vi "curvature to lookahead point.vi"(6 "Lookahead Distance":dbl, 11 "Path Data":T1={"Path"=[], "Target Velocities"=[], "Robot Location"=[], "Relative Robot Angle (rad)"=0.0, "Curvature"=0.0, "Lookahead Point"=[3064.399009129367, 18229.833030071386], "Lookahead Index"=8.422809037111724, "Closest Point"=[], "Closest Point Index"=0, "Left Velocity"=0.0, "Right Velocity"=0.0, "Left Encoder Vel"=0, "Right Encoder Vel"=0, "Left Encoder Pos"=0, "Right Encoder Pos"=0, "Inital Robot Angle (deg)"=0.0}) -> (3 "Path Data":T1={"Path"=[], "Target Velocities"=[], "Robot Location"=[], "Relative Robot Angle (rad)"=0.0, "Curvature"=0.0, "Lookahead Point"=[3064.399009129367, 18229.833030071386], "Lookahead Index"=8.422809037111724, "Closest Point"=[], "Closest Point Index"=0, "Left Velocity"=0.0, "Right Velocity"=0.0, "Left Encoder Vel"=0, "Right Encoder Vel"=0, "Left Encoder Pos"=0, "Right Encoder Pos"=0, "Inital Robot Angle (deg)"=0.0})   [LabVIEW 2018]
uses:
  path data.ctl
panel:
  out "Curvature":dbl
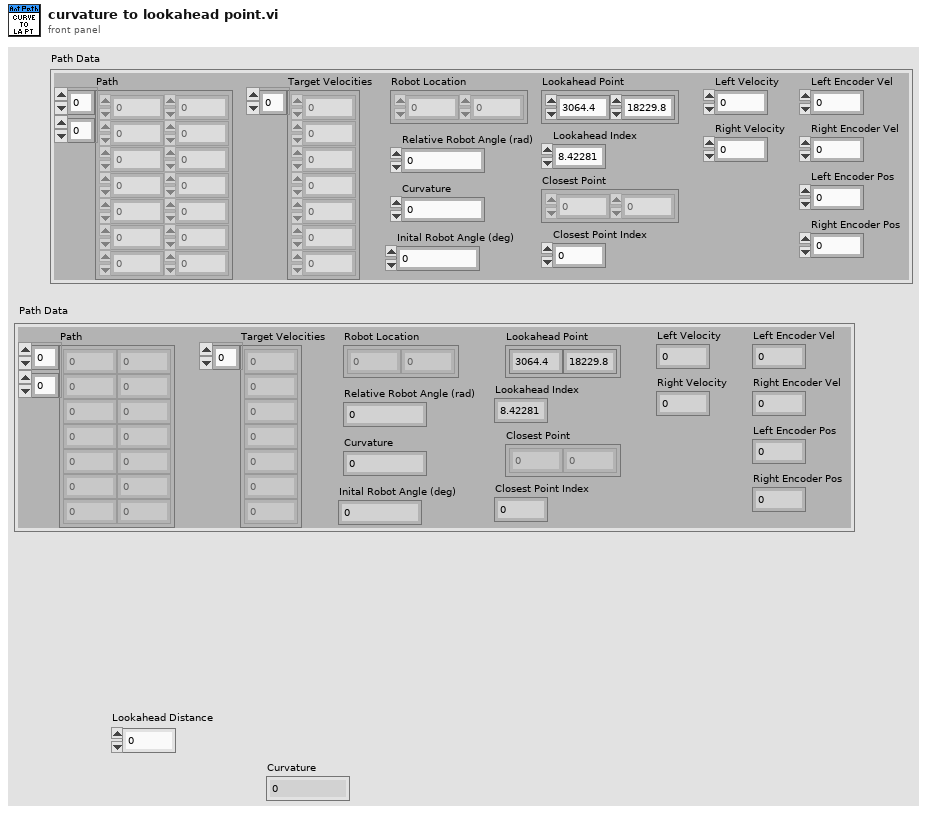
[diagram p1: front panel]
types:
  T1 = typedef "path data.ctl" = cluster{"Path":dbl[][], "Target Velocities":dbl[], "Robot Location":dbl[], "Relative Robot Angle (rad)":dbl, "Curvature":dbl, "Lookahead Point":dbl[], "Lookahead Index":dbl, "Closest Point":dbl[], "Closest Point Index":i32, "Left Velocity":dbl, "Right Velocity":dbl, "Left Encoder Vel":i32, "Right Encoder Vel":i32, "Left Encoder Pos":i32, "Right Encoder Pos":i32, "Inital Robot Angle (deg)":dbl}
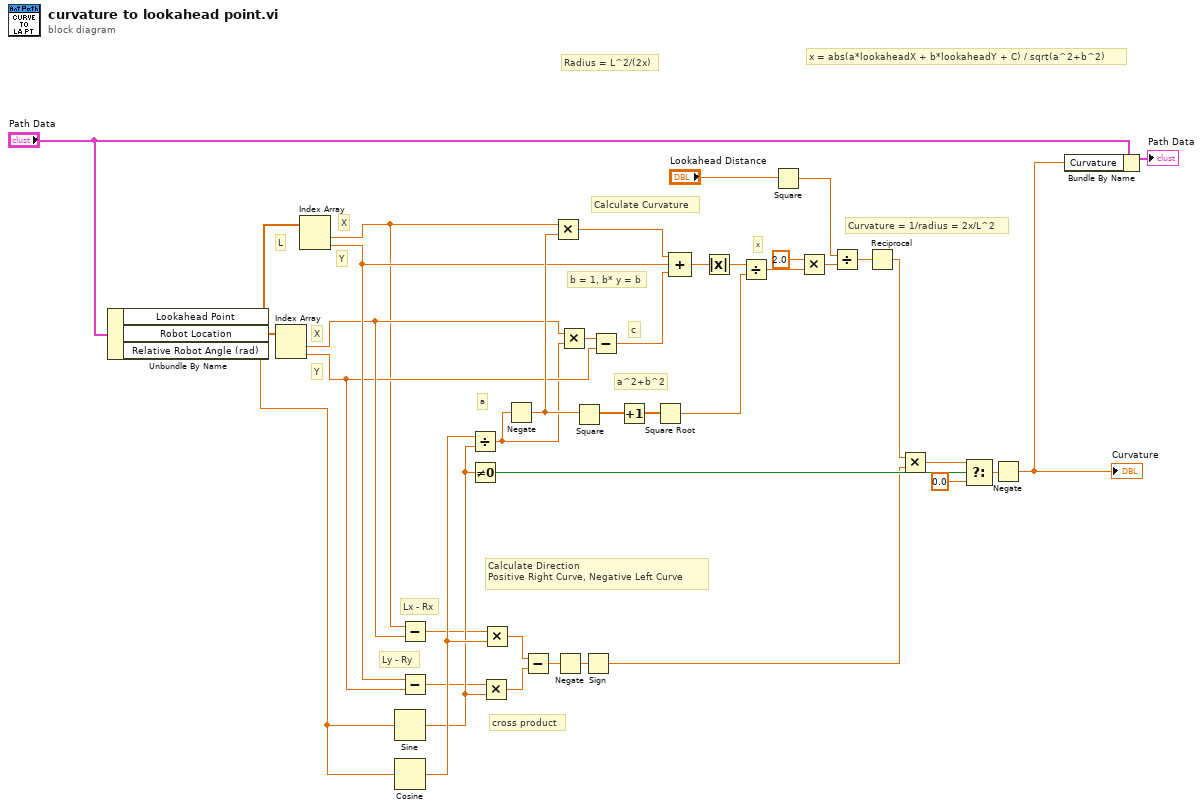
[diagram p0: block diagram]
diagram:
  # "cross product"
  # "Y"
  # "X"
  # "Y"
  # "X"
  # "Curvature = 1/radius = 2x/L^2"
  # "Calculate Direction\nPositive Right Curve, Negative Left Curve"
  # "Calculate Curvature"
  # "Ly - Ry"
  # "Lx - Rx"
  # "x"
  # "a^2+b^2"
  # "b = 1, b* y = b"
  # "x = abs(a*lookaheadX + b*lookaheadY + C) / sqrt(a^2+b^2)"
  # "a"
  # "c"
  # "L"
  # "Radius = L^2/(2x)"
  n1 = Unbundle By Name("Path Data") -> ("Lookahead Point"=w4:dbl[], "Robot Location"=w3:dbl[], "Relative Robot Angle (rad)"=w2:dbl)
  n2 = Index Array(array=w3) -> (element #1=w25:dbl, element #2=w24:dbl)  [unwired: 2 in]
  n3 = Index Array(array=w4) -> (element #1=w23:dbl, element #2=w26:dbl)  [unwired: 2 in]
  n4 = Sine(x=w2) -> (sin(x)=w19:dbl)
  n5 = Cosine(x=w2) -> (cos(x)=w20:dbl)
  n6 = Subtract(x=w23, y=w25) -> (x-y=w9:dbl)
  n7 = Subtract(x=w26, y=w24) -> (x-y=w8:dbl)
  n8 = Divide(x=w20, y=w19) -> (x/y=w18:dbl)
  n9 = Not Equal To 0?(x=w19) -> (x != 0?=w17:bool)
  n10 = Multiply(x=w8, y=w19) -> (x*y=w12:dbl)
  n11 = Multiply(x=w9, y=w20) -> (x*y=w13:dbl)
  n12 = Negate(x=w18) -> (-x=w36:dbl)
  n13 = Subtract(x=w13, y=w12) -> (x-y=w11:dbl)
  n14 = Multiply(x=w23, y=w36) -> (x*y=w39:dbl)
  n15 = Negate(x=w11) -> (-x=w10:dbl)
  n16 = Multiply(x=w25, y=w18) -> (x*y=w40:dbl)
  n17 = Square(x=w36) -> (x^2=w35:dbl)
  n18 = Sign(1:w10) -> (0:w14:dbl)
  n19 = Subtract(x=w40, y=w24) -> (x-y=w38:dbl)
  n20 = Increment(x=w35) -> (x+1=w34:dbl)
  n21 = Square Root(x=w34) -> (sqrt(x)=w33:dbl)
  n22 = Compound Arithmetic op=ADD(w39, w26, w38) -> (w37:dbl)
  n23 = Absolute Value(x=w37) -> (abs(x)=w32:dbl)
  n24 = Divide(x=w32, y=w33) -> (x/y=w30:dbl)
  n25 = Square(x="Lookahead Distance") -> (x^2=w29:dbl)
  n26 = Multiply(x=2.0, y=w30) -> (x*y=w22:dbl)
  n27 = Divide(x=w29, y=w22) -> (x/y=w28:dbl)
  n28 = Reciprocal(x=w28) -> (1/x=w27:dbl)
  n29 = Multiply(x=w27, y=w14) -> (x*y=w16:dbl)
  n30 = Select(t=w16, s=w17, f=0.0) -> (s? t:f=w5:dbl)
  n31 = Negate(x=w5) -> (-x=w1:dbl)
  "Curvature" <- w1
  n32 = Bundle By Name(cluster="Path Data", "Curvature"=w1) -> (→"Path Data":T1)
